vi "Host - TCP Engine.vi"() -> ()   [LabVIEW 2017]
uses:
  Controls/Read File.ctl
  Controls/Host- Queue States.ctl
  TCP Engine/Controls/TCP - Signals.ctl
  TCP Engine/Controls/TCP - Signal Names.ctl
  Controls/Control - Testscreen.ctl
  Controls/Test - Step Result.ctl
  Controls/Test details.ctl
  TCP Engine/Controls/TCP - Driver Control State.ctl
  Variable/Global 1.vi
  TCP Engine/Controls/TCP - Test Settings.ctl
  RT/Controls/RT- Get Set.ctl
panel:
  out "Log Path 2":path
  out "Log Path":path
  out "Waveform Chart":u32(graph)
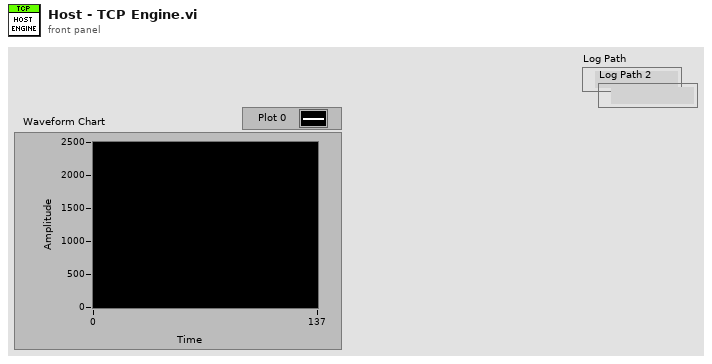
[diagram p1: front panel]
types:
  T1 = typedef "Host- Queue States.ctl" = enum16{"Initialize", "Enqueue", "Enqueue Priority", "Dequeue", "Flush", "Destroy"}
  T2 = typedef "Read File.ctl" = enum16{"Fetch XML", "Open", "Read", "Write", "Close"}
  T3 = typedef "TCP - Test Settings.ctl" = cluster{"Sequence File":string, "Iteration":i32}
  T4 = typedef "TCP - Signals.ctl" = cluster{"Signal":T5, "Value":bool, "Data":variant}
  T5 = typedef "TCP - Signal Names.ctl" = enum16{"Test Running", "Start Test", "Test Started", "Sequence Complete", "Seuence Aborted", "Abort Test", "Test Settings Updated", "Log Path", "Update Manual Values", "Start Aux Logging", "Aux Log Started", "Stop Aux Logging", "Aux Log Stopped", "Set Dyno Config", "Get PID Values", "Reset Emergency", "Copy Log File", "Download Files", "Send Test Details", "Generate Alarm"}
  T6 = typedef "Control - Testscreen.ctl" = enum16{"No Event", "Init", "Load Settings", "Save Setting", "Save Test Info", "Get Report", "Download Files", "Test Running", "Update Test Results", "Machine Unhealthy", "Autotest Started", "Test Aborted", "Sequence Complete", "Update Sensor Data", "Log File Available", "Machine Mode", "Aux Logging Started", "Aux File Saved", "Get PID Values", "View Report", "Exit", "Wait", "Abort", "Copy Log File", "Generate Alarm", "Send Test Details"}
  T7 = typedef "Test - Step Result.ctl" = cluster{"Step Name":string, "Value":dbl, "Success ?":bool, "Stop Seq ?":bool, "Abort":bool, "Sr.No":i32}
  T8 = typedef "RT- Get Set.ctl" = enum16{"Reset", "Get", "Set"}
  T9 = typedef "Test details.ctl" = cluster{"Furnace":string, "Material":string, "Angle":string, "ID":string, "Flowrate":string, "Test Name":string, "Tested By":string}
  T10 = typedef "TCP - Driver Control State.ctl" = enum16{"Test Settings", "Send Test Details", "Boolean Commands", "Test Results"}
  T11 = typedef "TCP - Driver control.ctl" = enum16{"Test Settings", "Boolean Commands", "Test Results", "Send Test Details"}
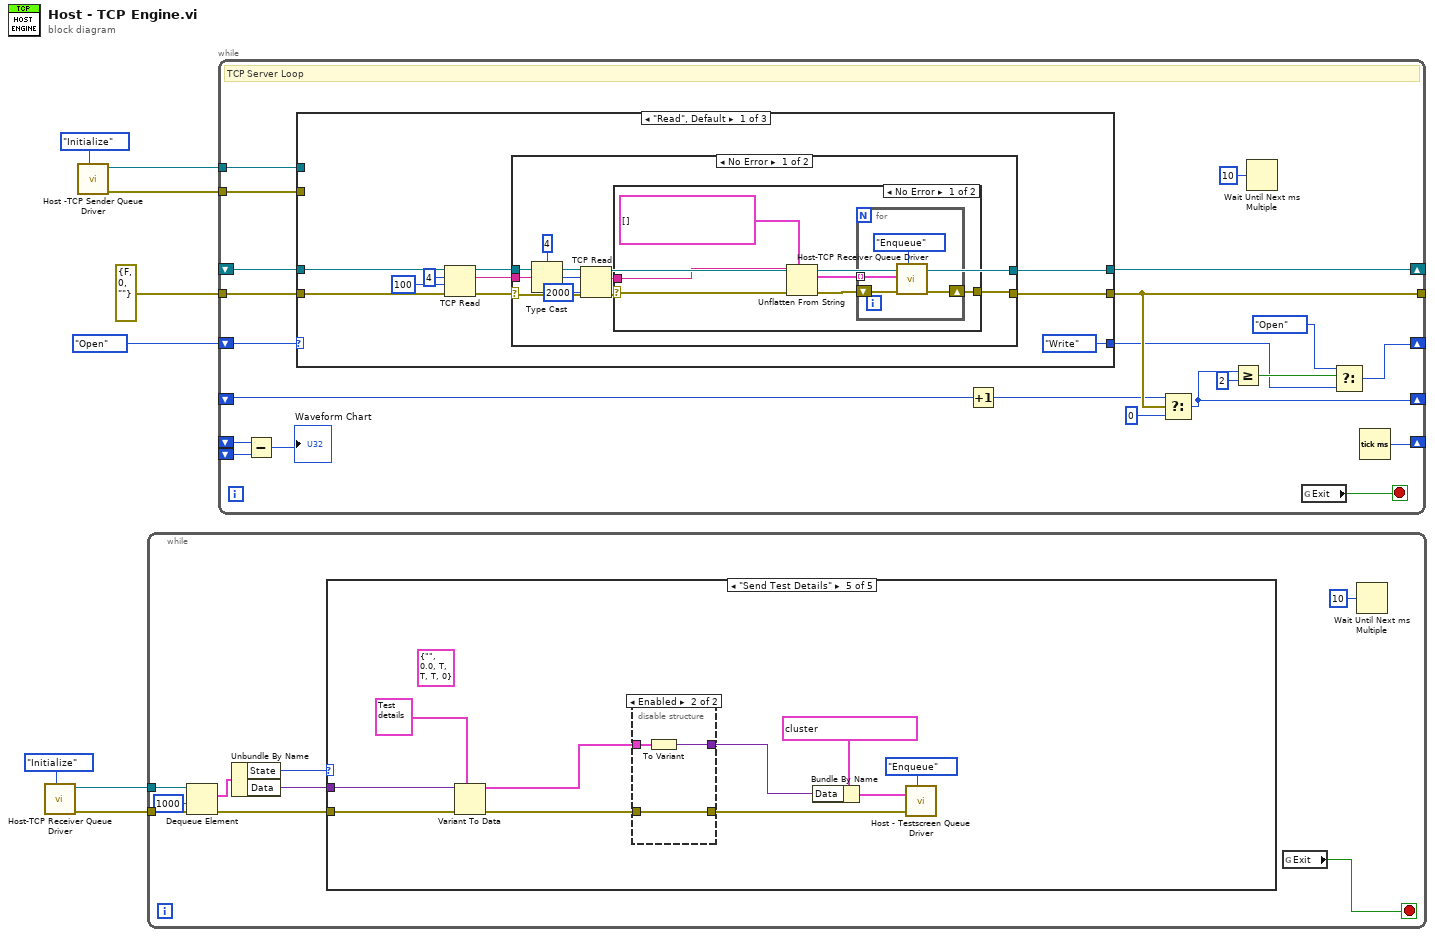
[diagram p0: block diagram]
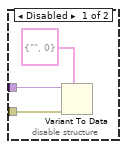
[diagram p3: hidden frame]
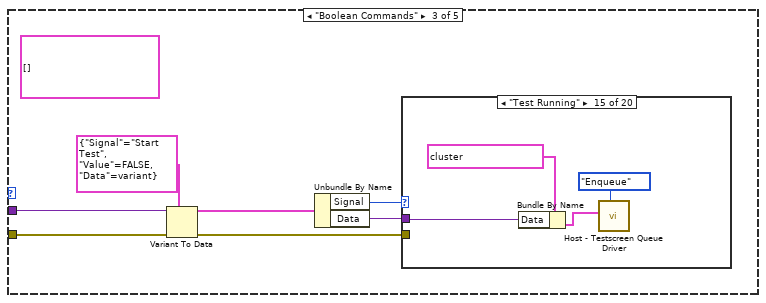
[diagram p5: hidden frame]
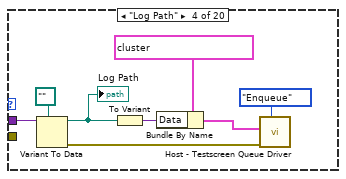
[diagram p9: hidden frame]
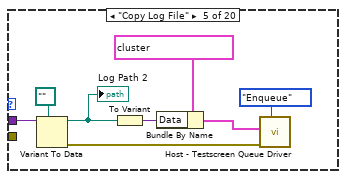
[diagram p10: hidden frame]
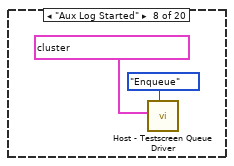
[diagram p13: hidden frame]
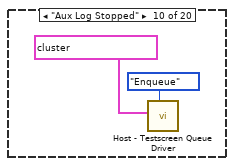
[diagram p15: hidden frame]
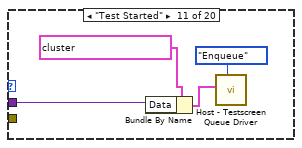
[diagram p16: hidden frame]
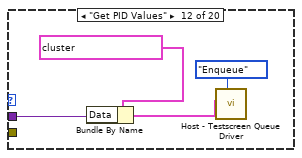
[diagram p17: hidden frame]
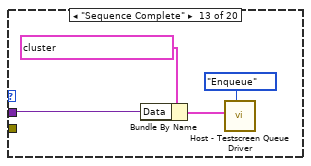
[diagram p18: hidden frame]
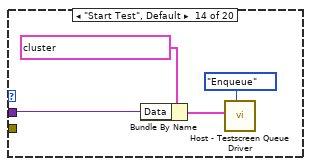
[diagram p19: hidden frame]
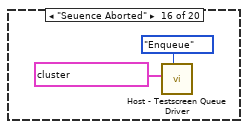
[diagram p20: hidden frame]
diagram:
  n1 = call "Host-TCP Receiver Queue Driver.vi"("Cases"=Host-_Queue_States."Initialize") -> ("error out"=w5:errorcluster, "queue out"=w6:refnum<queue>)  [unwired: 8 in, 1 out]
  n2 = call "Host -TCP Sender Queue Driver.vi"("Cases"=Host-_Queue_States."Initialize") -> ("error out"=w1:errorcluster, "queue out"=w2:refnum<queue>)  [unwired: 8 in, 1 out]
  n3 = while {
    tunnel: w6 -> [w16]
    tunnel: w5 -> [w17]
    stop <- w9 stop-if-true
    n4 = Dequeue Element(queue=w16, timeout in ms (-1)=1000, error in (no error)=w17) -> (element=w14:cluster{"Data":variant, "State":T10}, error out=w15:errorcluster)  [unwired: 2 out]
    n5 = Unbundle By Name(w14) -> ("State"=w12:T10, "Data"=w11:variant)
    n6 = case shown="\"Send Test Details\"" w12 {
      tunnel: w15 -> [w19 _ w28 w84 w101]
      tunnel: w11 -> [w18 _ w29 w85 w102]
      frame "Test Settings" {
        n7 = disable-structure shown="Enabled" {
          disable-tunnel: w19 -> [w22 _]
          disable-tunnel: w18 -> [w21 _]
          frame Disabled {
            n8 = Variant To Data(error in=w22, type=T3 {"Sequence File"="", "Iteration"=0}, Variant=w21) -> ()  [unwired: 2 out]
          }
          frame Enabled {
          }
        }
      }
      frame Default {
      }
      frame "Boolean Commands" {
        (unwired) T4[] [] ("Array")
        n9 = Variant To Data(error in=w28, type=T4 {"Signal"=enum."Start Test", "Value"=FALSE, "Data"=variant}, Variant=w29) -> (data=w26:T4, error out=w23:errorcluster)
        n10 = Unbundle By Name(w26) -> ("Signal"=w25:T5, "Data"=w24:variant)
        n11 = case shown="\"Test Running\"" w25 {
          tunnel: w24 -> [_ _ _ w37 w45 _ _ _ _ _ w52 w55 w60 w64 w68 _ w72 _ _ _]
          tunnel: w23 -> [_ _ _ _ _ _ _ _ _ _ _ _ _ _ _ _ _ _ _ _]
          frame "Abort Test" {
          }
          frame "Test Settings Updated" {
          }
          frame "Set Dyno Config" {
          }
          frame "Log Path" {
            n12 = Variant To Data(type=path "", Variant=w37) -> (data=w32:path, error out=w34:errorcluster)  [unwired: 1 in]
            "Log Path" <- w32
            n13 = To Variant(anything=w32) -> (Variant=w31:variant)
            n14 = Bundle By Name(cluster=cluster{"Data":variant, "Enum":T6} {"Data"=variant, "Enum"=enum."Log File Available"} ("Element In"), "Data"=w31) -> (w30:cluster{"Data":variant, "Enum":T6})
            n15 = call "Host - Testscreen Queue Driver.vi"("Cases"=Host-_Queue_States."Enqueue", "error in (no error)"=w34, "Element In"=w30) -> ()  [unwired: 6 in, 3 out]
          }
          frame "Copy Log File" {
            n16 = Variant To Data(type=path "", Variant=w45) -> (data=w40:path, error out=w42:errorcluster)  [unwired: 1 in]
            "Log Path 2" <- w40
            n17 = To Variant(anything=w40) -> (Variant=w39:variant)
            n18 = Bundle By Name(cluster=cluster{"Data":variant, "Enum":T6} {"Data"=variant, "Enum"=enum."Copy Log File"} ("Element In"), "Data"=w39) -> (w38:cluster{"Data":variant, "Enum":T6})
            n19 = call "Host - Testscreen Queue Driver.vi"("Cases"=Host-_Queue_States."Enqueue", "error in (no error)"=w42, "Element In"=w38) -> ()  [unwired: 6 in, 3 out]
          }
          frame "Update Manual Values" {
          }
          frame "Start Aux Logging" {
          }
          frame "Aux Log Started" {
            n20 = call "Host - Testscreen Queue Driver.vi"("Cases"=Host-_Queue_States."Enqueue", "Element In"=cluster{"Data":variant, "Enum":T6} {"Data"=variant, "Enum"=enum."Aux Logging Started"}) -> ()  [unwired: 7 in, 3 out]
          }
          frame "Stop Aux Logging" {
          }
          frame "Aux Log Stopped" {
            n21 = call "Host - Testscreen Queue Driver.vi"("Cases"=Host-_Queue_States."Enqueue", "Element In"=cluster{"Data":variant, "Enum":T6} {"Data"=variant, "Enum"=enum."Aux File Saved"}) -> ()  [unwired: 7 in, 3 out]
          }
          frame "Test Started" {
            n22 = Bundle By Name(cluster=cluster{"Data":variant, "Enum":T6} {"Data"=variant, "Enum"=enum."Autotest Started"} ("Element In"), "Data"=w52) -> (w50:cluster{"Data":variant, "Enum":T6})
            n23 = call "Host - Testscreen Queue Driver.vi"("Cases"=Host-_Queue_States."Enqueue", "Element In"=w50) -> ()  [unwired: 7 in, 3 out]
          }
          frame "Get PID Values" {
            n24 = Bundle By Name(cluster=cluster{"Data":variant, "Enum":T6} {"Data"=variant, "Enum"=enum."Get PID Values"} ("Element In"), "Data"=w55) -> (w54:cluster{"Data":variant, "Enum":T6})
            n25 = call "Host - Testscreen Queue Driver.vi"("Cases"=Host-_Queue_States."Enqueue", "Element In"=w54) -> ()  [unwired: 7 in, 3 out]
          }
          frame "Sequence Complete" {
            n26 = Bundle By Name(cluster=cluster{"Data":variant, "Enum":T6} {"Data"=variant, "Enum"=enum."Sequence Complete"} ("Element In"), "Data"=w60) -> (w58:cluster{"Data":variant, "Enum":T6})
            n27 = call "Host - Testscreen Queue Driver.vi"("Cases"=Host-_Queue_States."Enqueue", "Element In"=w58) -> ()  [unwired: 7 in, 3 out]
          }
          frame "Start Test", Default {
            n28 = Bundle By Name(cluster=cluster{"Data":variant, "Enum":T6} {"Data"=variant, "Enum"=enum."Update Sensor Data"} ("Element In"), "Data"=w64) -> (w62:cluster{"Data":variant, "Enum":T6})
            n29 = call "Host - Testscreen Queue Driver.vi"("Cases"=Host-_Queue_States."Enqueue", "Element In"=w62) -> ()  [unwired: 7 in, 3 out]
          }
          frame "Test Running" {
            n30 = Bundle By Name(cluster=cluster{"Data":variant, "Enum":T6} {"Data"=variant, "Enum"=enum."Test Running"} ("Element In"), "Data"=w68) -> (w66:cluster{"Data":variant, "Enum":T6})
            n31 = call "Host - Testscreen Queue Driver.vi"("Cases"=Host-_Queue_States."Enqueue", "Element In"=w66) -> ()  [unwired: 7 in, 3 out]
          }
          frame "Seuence Aborted" {
            n32 = call "Host - Testscreen Queue Driver.vi"("Cases"=Host-_Queue_States."Enqueue", "Element In"=cluster{"Data":variant, "Enum":T6} {"Data"=variant, "Enum"=enum."Test Aborted"}) -> ()  [unwired: 7 in, 3 out]
          }
          frame "Generate Alarm" {
            n33 = Bundle By Name(cluster=cluster{"Data":variant, "Enum":T6} {"Data"=variant, "Enum"=enum."Generate Alarm"} ("Element In"), "Data"=w72) -> (w73:cluster{"Data":variant, "Enum":T6})
            n34 = call "Host - Testscreen Queue Driver.vi"("Cases"=Host-_Queue_States."Enqueue", "Element In"=w73) -> ()  [unwired: 7 in, 3 out]
          }
          frame "Reset Emergency" {
          }
          frame "Download Files" {
          }
          frame "Send Test Details" {
          }
        }
      }
      frame "Test Results" {
        n35 = Variant To Data(error in=w84, type=T7 {"Step Name"="", "Value"=0.0, "Success ?"=TRUE, "Stop Seq ?"=TRUE, "Abort"=TRUE, "Sr.No"=0} ("element"), Variant=w85) -> (data=w81:T7, error out=w80:errorcluster)
        n36 = disable-structure shown="Enabled" {
          disable-tunnel: w81 -> [w88 w92]
          disable-tunnel: w80 -> [w87 w91]
          disable-tunnel: [w86 w91] -> w79
          disable-tunnel: [_ w90] -> w77
          frame Disabled {
            n37 = call "Test - FGV - Test Results.vi"("Get/Set"=RT-_Get_Set."Set", "error in (no error)"=w87, "Step Result"=w88) -> ("error out"=w86:errorcluster)  [unwired: 7 in, 1 out]
          }
          frame Enabled {
            n38 = To Variant(anything=w92) -> (Variant=w90:variant)
          }
        }
        n39 = Bundle By Name(cluster=cluster{"Data":variant, "Enum":T6} {"Data"=variant, "Enum"=enum."Update Test Results"} ("Element In"), "Data"=w77) -> (w76:cluster{"Data":variant, "Enum":T6})
        n40 = call "Host - Testscreen Queue Driver.vi"("Cases"=Host-_Queue_States."Enqueue", "error in (no error)"=w79, "Element In"=w76) -> ()  [unwired: 6 in, 3 out]
      }
      frame "Send Test Details" {
        (unwired) T7 {"Step Name"="", "Value"=0.0, "Success ?"=TRUE, "Stop Seq ?"=TRUE, "Abort"=TRUE, "Sr.No"=0} ("element")
        n41 = Variant To Data(error in=w101, type=T9 {"Furnace"="Furnace A", "Material"="Coke", "Angle"="Multi Angle", "ID"="Trajectory 9", "Flowrate"="Flow", "Test Name"="Coke Burn", "Tested By"="Anirban"} ("Test details"), Variant=w102) -> (data=w99:T9, error out=w98:errorcluster)
        n42 = disable-structure shown="Enabled" {
          disable-tunnel: w99 -> [w105 w109]
          disable-tunnel: w98 -> [w104 w108]
          disable-tunnel: [w103 w108] -> w97
          disable-tunnel: [_ w107] -> w95
          frame Disabled {
            n43 = call "Test - FGV - Test Results.vi"("Get/Set"=RT-_Get_Set."Set", "error in (no error)"=w104, "Step Result"=w105) -> ("error out"=w103:errorcluster)  [unwired: 7 in, 1 out]
          }
          frame Enabled {
            n44 = To Variant(anything=w109) -> (Variant=w107:variant)
          }
        }
        n45 = Bundle By Name(cluster=cluster{"Data":variant, "Enum":T6} {"Data"=variant, "Enum"=enum."Send Test Details"} ("Element In"), "Data"=w95) -> (w94:cluster{"Data":variant, "Enum":T6})
        n46 = call "Host - Testscreen Queue Driver.vi"("Cases"=Host-_Queue_States."Enqueue", "error in (no error)"=w97, "Element In"=w94) -> ()  [unwired: 6 in, 3 out]
      }
    }
    n47 = global read "Global 1.vi" "Exit"() -> (w9:bool)
    n48 = Wait Until Next ms Multiple(millisecond multiple=u32 10) -> ()  [unwired: 1 out]
  }
  n49 = while {
    shift-right: [w130] -> _
    shift-left: _ -> [w129]
    shift-right: [w120] -> _
    shift-left: Read_File."Open" ("R/W") -> [w131]
    shift-right: [w123] -> _
    shift-left: _ -> [w125]
    tunnel: w2 -> [w118]
    tunnel: w1 -> [w117]
    tunnel: errorcluster {"status"=FALSE, "code"=0, "source"=""} ("error out") -> [w128]
    tunnel: [w127] -> _
    shift-right: [w114] -> _
    shift-left: _ -> [w113]
    shift-left: _ -> [w112]
    stop <- w110 stop-if-true
    # "TCP Server Loop"
    n50 = Subtract(x=w113, y=w112) -> (x-y=→"Waveform Chart":u32)
    n51 = case shown="\"Read\", Default" w131 {
      tunnel: [w136 w179 w195] -> w130
      tunnel: [w135 w178 w194] -> w127
      tunnel: w129 -> [w141 w167 _]
      tunnel: w128 -> [w140 w170 _]
      tunnel: [Read_File."Write" ("R/W") Read_File."Read" ("R/W") w196] -> w116
      tunnel: w118 -> [_ w172 _]
      tunnel: w117 -> [_ w171 _]
      frame "Read", Default {
        n52 = TCP Read(connection ID=w141, bytes to read=4, error in (no error)=w140, 9:100 ("timeout ms (25000)")) -> (connection ID out=w139:refnum<k5>, data out=w134:string, error out=w132:errorcluster)  [unwired: 1 out]
        n53 = case shown="No Error" w132 {
          selector: w132 -> [w146 w163]
          tunnel: w139 -> [w151 w164]
          tunnel: [w150 w164] -> w136
          tunnel: [w145 w163] -> w135
          tunnel: w134 -> [w148 _]
          frame No Error {
            n54 = Type Cast(type=4 ("bytes to read"), x=w148) -> (*(type *) &x=w147:i32)
            n55 = TCP Read(connection ID=w151, bytes to read=w147, error in (no error)=w146, 9:2000 ("timeout ms (25000)")) -> (connection ID out=w150:refnum<k5>, data out=w144:string, error out=w143:errorcluster)  [unwired: 1 out]
            n56 = case shown="No Error" w143 {
              selector: w143 -> [w154 w162]
              tunnel: w144 -> [w155 _]
              tunnel: [w157 w162] -> w145
              frame No Error {
                n57 = Unflatten From String(type=cluster{"Data":variant, "State":T10}[] [], binary string=w155, error in (no error)=w154) -> (value=w152:cluster{"Data":variant, "State":T10}[], error out=w153:errorcluster)  [unwired: 2 in, 1 out]
                n58 = for {
                  tunnel: w152 -> [w159] mode=indexing
                  shift-right: [w161] -> w157
                  shift-left: w153 -> [w160]
                  n59 = call "Host-TCP Receiver Queue Driver.vi"("Cases"=Host-_Queue_States."Enqueue", "error in (no error)"=w160, "Element In"=w159) -> ("error out"=w161:errorcluster)  [unwired: 6 in, 2 out]
                }
              }
              frame Error {
              }
            }
          }
          frame Error {
          }
        }
      }
      frame "Write" {
        n60 = Get Queue Status(queue=w172, return elements? (F)=TRUE, error in (no error)=w171) -> (queue out=w165:refnum<queue>, elements=w174:cluster{"Data":variant, "State":T11}[])  [unwired: 6 out]
        n61 = Flatten To String(anything=w174, error in (no error)=w170) -> (data string=w166:string, error out=w169:errorcluster)  [unwired: 2 in, 1 out]
        n62 = String Length(string=w166) -> (length=w175:i32)
        n63 = Type Cast(x=w175) -> (*(type *) &x=w168:string)  [unwired: 1 out]
        n64 = TCP Write(connection ID=w167, data in=w168, error in (no error)=w169, 9:100 ("timeout ms (25000)")) -> (connection ID out=w180:refnum<k5>, error out=w176:errorcluster)  [unwired: 1 out]
        n65 = case shown="No Error" w176 {
          selector: w176 -> [w185 w189]
          tunnel: w180 -> [w188 w190]
          tunnel: [w187 w190] -> w179
          tunnel: [w186 w189] -> w178
          tunnel: w166 -> [_ _]
          tunnel: w165 -> [w184 _]
          frame No Error {
            n66 = Flush Queue(queue=w184) -> (remaining elements=w183:cluster{"Data":variant, "State":T11}[])  [unwired: 1 in, 2 out]
            n67 = Empty Array?(array=w183) -> ()  [unwired: 1 out]
            n68 = Flatten To String(anything=w183) -> (data string=w182:string)  [unwired: 3 in, 2 out]
            n69 = TCP Write(connection ID=w188, data in=w182, error in (no error)=w185) -> (connection ID out=w187:refnum<k5>, error out=w186:errorcluster)  [unwired: 2 out]
          }
          frame Error {
          }
        }
      }
      frame "Open" {
        (unwired) "localhost" ("address")
        (unwired) "192.168.0.3" ("address")
        w192 = u16 6340  # port
        w193 = 2000  # timeout (ms)
        n70 = TCP Open Connection(address="169.254.10.138" ("service name"), remote port or service name=w192, timeout ms (60000)=w193) -> (connection ID=w195:refnum<k5>, error out=w194:errorcluster)  [unwired: 2 in]
        n71 = Select(t=Read_File."Open", s=w194, f=Read_File."Read" ("R/W")) -> (s? t:f=w196:T2)
      }
    }
    n72 = Increment(x=w125) -> (x+1=w124:i32)
    n73 = Select(t=w124, s=w127, f=0) -> (s? t:f=w123:i32)
    n74 = Greater Or Equal?(x=w123, y=2) -> (x >= y?=w121:bool)
    n75 = Wait Until Next ms Multiple(millisecond multiple=u32 10) -> ()  [unwired: 1 out]
    n76 = global read "Global 1.vi" "Exit"() -> (w110:bool)
    n77 = Select(t=Read_File."Open" ("f"), s=w121, f=w116) -> (s? t:f=w120:T2)
    n78 = Tick Count (ms)() -> (millisecond timer value=w114:u32)
  }
